vi "Check Status of Home Routine.vi"(8 "error in (no error)":errorcluster, 11 "Fine SIM Motion Controller in":refnum<class "Fine SIM Motion Controller.lvclass">) -> (0 "error out":errorcluster, 3 "Fine SIM Motion Controller out":refnum<class "Fine SIM Motion Controller.lvclass">)   [LabVIEW 2022 SP3, in "Fine SIM Motion Controller.lvclass"]
uses:
  Fine SIM Motion Controller.lvclass
  C:/Stage-Work/MAS/Axis Objects/Motion Controller/Parent SIM Motion Controller.lvclass
  Motion Controller/Parent SIM Motion Controller.lvclass/Parent SIM Motion Controller.ctl
  Motion Controller/Homing Status.ctl
  Motion Controller/Accessors/Read Sim Axis Data.vi
  Motion Controller/Accessors/Write Sim Axis Data.vi
  Fine SIM Motion Controller.lvclass/Fine SIM Motion Controller.ctl
  Motion Controller/Parent SIM Motion Controller.lvclass
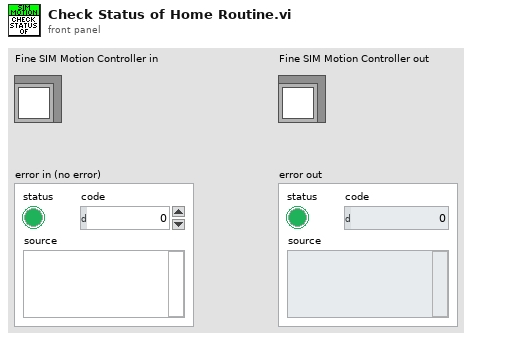
[diagram p1: front panel]
types:
  T1 = typedef "Parent SIM Motion Controller.lvclass/Axis Data.ctl" = cluster{"Axis Parameters":T2, "Axis Settings":T4, "Time Stamp":timestamp}
  T2 = typedef "Parent SIM Motion Controller.lvclass/Axis Parameters.ctl" = cluster{"Moving":bool, "Homed":bool, "Desired Position":dbl, "Current Positon":dbl, "Current Speed":dbl, "Home Status":T3}
  T3 = typedef "Parent SIM Motion Controller.lvclass/Homing Status.ctl" = enum16{"Idle", "Inital Home Motion", "Final Home Motion", "Done Homing"}
  T4 = typedef "Parent SIM Motion Controller.lvclass/Axis Settings.ctl" = cluster{"Speed":dbl, "Acceleration":dbl}
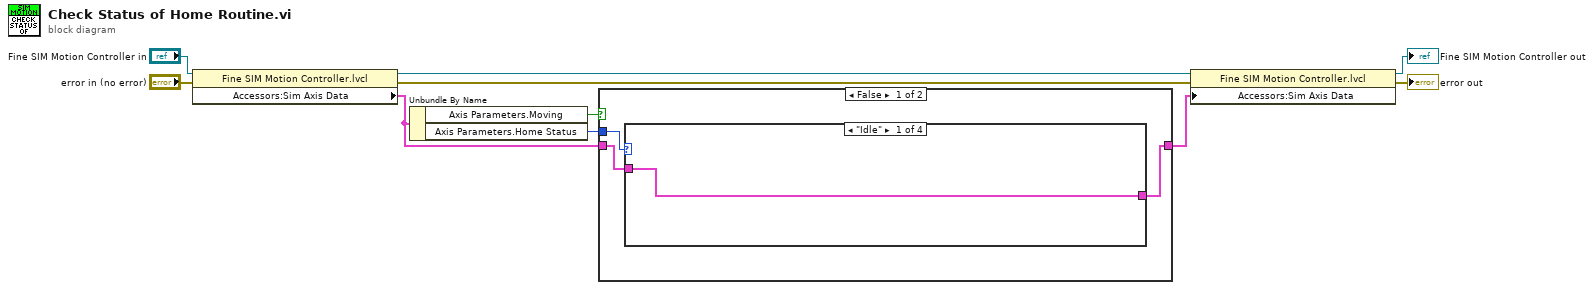
[diagram p0: block diagram]
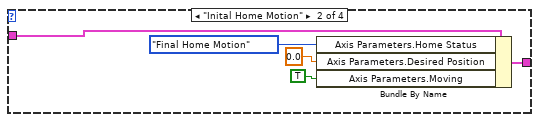
[diagram p2: hidden frame]
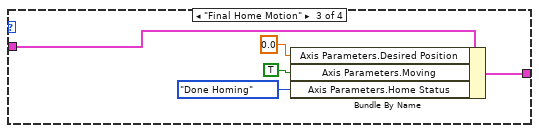
[diagram p3: hidden frame]
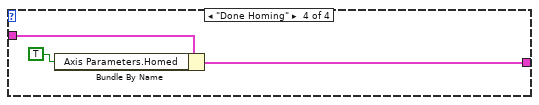
[diagram p4: hidden frame]
diagram:
  n1 = property class="Fine SIM Motion Controller.lvcl"(reference="Fine SIM Motion Controller in", error in="error in (no error)") -> (reference out=w4:refnum<class "Fine SIM Motion Controller.lvclass">, error out=w8:errorcluster, "Accessors:Sim Axis Data"=w1:T1)
  n2 = Unbundle By Name(w1) -> ("Axis Parameters.Moving"=w6:bool, "Axis Parameters.Home Status"=w9:T3)
  n3 = case shown="False" w6 {
    tunnel: w9 -> [w11 _]
    tunnel: [w13 w28] -> w2
    tunnel: w1 -> [w12 w28]
    frame False {
      n4 = case shown="\"Idle\"" w11 {
        tunnel: [w14 w18 w23 w27] -> w13
        tunnel: w12 -> [w14 w15 w21 w26]
        frame "Idle" {
        }
        frame "Inital Home Motion" {
          n5 = Bundle By Name(cluster=w15, "Axis Parameters.Home Status"=Homing_Status."Final Home Motion", "Axis Parameters.Desired Position"=0.0, "Axis Parameters.Moving"=TRUE) -> (w18:T1)
        }
        frame "Final Home Motion" {
          n6 = Bundle By Name(cluster=w21, "Axis Parameters.Desired Position"=0.0, "Axis Parameters.Moving"=TRUE, "Axis Parameters.Home Status"=Homing_Status."Done Homing") -> (w23:T1)
        }
        frame "Done Homing" {
          n7 = Bundle By Name(cluster=w26, "Axis Parameters.Homed"=TRUE) -> (w27:T1)
        }
      }
    }
    frame True {
    }
  }
  n8 = property class="Fine SIM Motion Controller.lvcl"(reference=w4, error in=w8, "Accessors:Sim Axis Data"=w2) -> (reference out=→"Fine SIM Motion Controller out":refnum<class "Fine SIM Motion Controller.lvclass">, error out=→"error out":errorcluster)
